vi "Update Status.vi"(7 "Check overlay?":bool, 8 "error in (no error)":errorcluster, 9 "Status":T1=enum."Passed", 10 "Case":string, 11 "Icon Decorator In":refnum<class "Icon Decorator.lvclass">) -> (0 "error out":errorcluster)   [LabVIEW 2020, in "Icon Decorator.lvclass"]
uses:
  Icon Decorator.lvclass
  Core/Result/Status.ctl
  Icon Decorator.lvclass/Icon Decorator.ctl
  <resource>/Framework/Providers/API/mxLvUpdateUI.ctl
  <resource>/Framework/Providers/API/mxLvOverlayState.ctl
  Core/Result/Result.lvlib
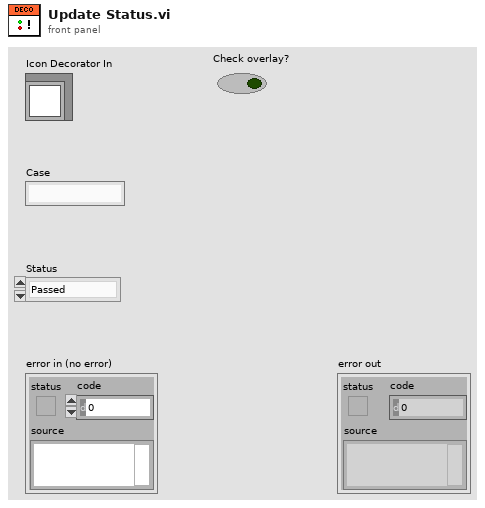
[diagram p1: front panel]
types:
  T1 = typedef "Result.lvlib/Status.ctl" = enum16{"", "Passed", "Failed", "Error", "Skipped", "Setup Error", "Broken", "Teardown Error"}
  T2 = typedef "ItemRef.ctl" = u64
  T3 = typedef "mxLvUpdateUI.ctl" = cluster{"Action":u32, "Optional param 1":string, "Optional param 2":i32, "Optional param 3":string}
  T4 = typedef "mxLvOverlayState.ctl" = cluster{"Overlay Alias":string, "Active":bool}
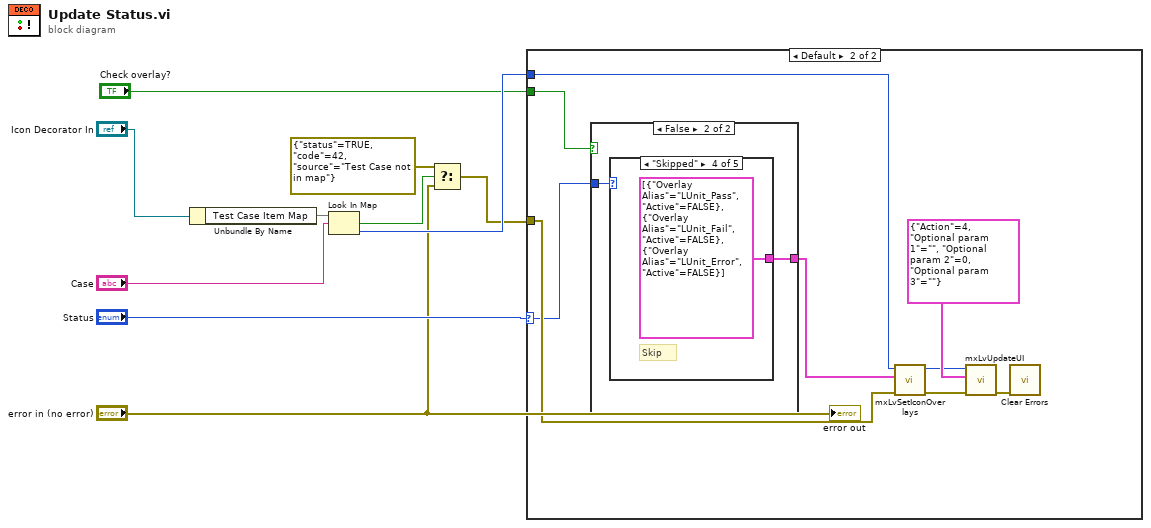
[diagram p0: block diagram]
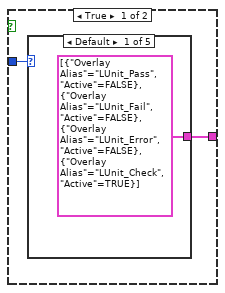
[diagram p3: hidden frame]
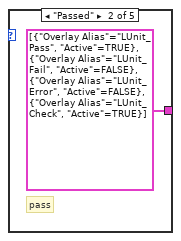
[diagram p4: hidden frame]
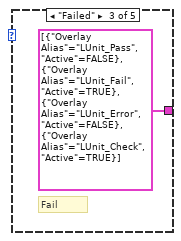
[diagram p5: hidden frame]
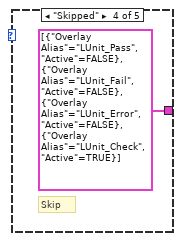
[diagram p6: hidden frame]
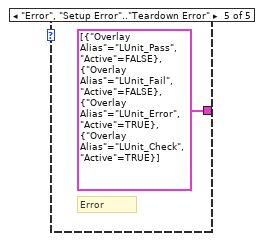
[diagram p7: hidden frame]
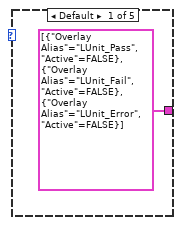
[diagram p8: hidden frame]
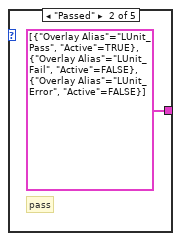
[diagram p9: hidden frame]
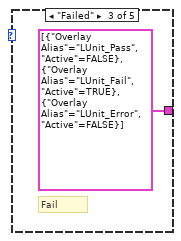
[diagram p10: hidden frame]
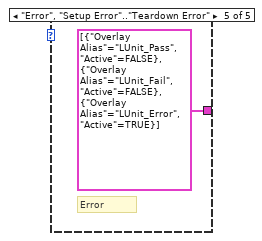
[diagram p11: hidden frame]
diagram:
  n1 = Unbundle By Name("Icon Decorator In") -> ("Test Case Item Map"=w1:map{string, T2})
  n2 = Look In Map(map=w1, key="Case") -> (key not found?=w2:bool, value=w7:T2)  [unwired: 1 in]
  n3 = Select(t=errorcluster {"status"=TRUE, "code"=42, "source"="Test Case not in map"}, s=w2, f="error in (no error)") -> (s? t:f=w6:errorcluster)
  n4 = case shown="Default" "Status" {
    selector: "Status" -> [_ w16]
    tunnel: w7 -> [_ w19]
    tunnel: w6 -> [_ w18]
    tunnel: "Check overlay?" -> [_ w15]
    frame "" {
    }
    frame Default {
      n5 = case shown="False" w15 {
        tunnel: w16 -> [w21 w28]
        tunnel: [w20 w27] -> w14
        frame True {
          n6 = case shown="Default" w21 {
            tunnel: [T4[] [{"Overlay Alias"="LUnit_Pass", "Active"=FALSE}, {"Overlay Alias"="LUnit_Fail", "Active"=FALSE}, {"Overlay Alias"="LUnit_Error", "Active"=FALSE}, {"Overlay Alias"="LUnit_Check", "Active"=TRUE}] ("Array") T4[] [{"Overlay Alias"="LUnit_Pass", "Active"=TRUE}, {"Overlay Alias"="LUnit_Fail", "Active"=FALSE}, {"Overlay Alias"="LUnit_Error", "Active"=FALSE}, {"Overlay Alias"="LUnit_Check", "Active"=TRUE}] ("Array") T4[] [{"Overlay Alias"="LUnit_Pass", "Active"=FALSE}, {"Overlay Alias"="LUnit_Fail", "Active"=TRUE}, {"Overlay Alias"="LUnit_Error", "Active"=FALSE}, {"Overlay Alias"="LUnit_Check", "Active"=TRUE}] ("Array") T4[] [{"Overlay Alias"="LUnit_Pass", "Active"=FALSE}, {"Overlay Alias"="LUnit_Fail", "Active"=FALSE}, {"Overlay Alias"="LUnit_Error", "Active"=FALSE}, {"Overlay Alias"="LUnit_Check", "Active"=TRUE}] ("Array") T4[] [{"Overlay Alias"="LUnit_Pass", "Active"=FALSE}, {"Overlay Alias"="LUnit_Fail", "Active"=FALSE}, {"Overlay Alias"="LUnit_Error", "Active"=TRUE}, {"Overlay Alias"="LUnit_Check", "Active"=TRUE}] ("Array")] -> w20
            frame Default {
            }
            frame "Passed" {
              # "pass"
            }
            frame "Failed" {
              # "Fail"
            }
            frame "Skipped" {
              # "Skip"
            }
            frame "Error", "Setup Error".."Teardown Error" {
              # "Error"
            }
          }
        }
        frame False {
          n7 = case shown="\"Skipped\"" w28 {
            tunnel: [T4[] [{"Overlay Alias"="LUnit_Pass", "Active"=FALSE}, {"Overlay Alias"="LUnit_Fail", "Active"=FALSE}, {"Overlay Alias"="LUnit_Error", "Active"=FALSE}] ("Array") T4[] [{"Overlay Alias"="LUnit_Pass", "Active"=TRUE}, {"Overlay Alias"="LUnit_Fail", "Active"=FALSE}, {"Overlay Alias"="LUnit_Error", "Active"=FALSE}] ("Array") T4[] [{"Overlay Alias"="LUnit_Pass", "Active"=FALSE}, {"Overlay Alias"="LUnit_Fail", "Active"=TRUE}, {"Overlay Alias"="LUnit_Error", "Active"=FALSE}] ("Array") T4[] [{"Overlay Alias"="LUnit_Pass", "Active"=FALSE}, {"Overlay Alias"="LUnit_Fail", "Active"=FALSE}, {"Overlay Alias"="LUnit_Error", "Active"=FALSE}] ("Array") T4[] [{"Overlay Alias"="LUnit_Pass", "Active"=FALSE}, {"Overlay Alias"="LUnit_Fail", "Active"=FALSE}, {"Overlay Alias"="LUnit_Error", "Active"=TRUE}] ("Array")] -> w27
            frame Default {
            }
            frame "Passed" {
              # "pass"
            }
            frame "Failed" {
              # "Fail"
            }
            frame "Skipped" {
              # "Skip"
            }
            frame "Error", "Setup Error".."Teardown Error" {
              # "Error"
            }
          }
        }
      }
      n8 = call <resource>:"mxLvSetIconOverlays.vi"("error in"=w18, "Overlay States"=w14, "Item"=w19) -> ("error out"=w11:errorcluster, "Item"=w12:T2)  [unwired: 7 in]
      n9 = call <resource>:"mxLvUpdateUI.vi"("error in"=w11, "Update UI Settings"=T3 {"Action"=4, "Optional param 1"="", "Optional param 2"=0, "Optional param 3"=""}, "Item"=w12) -> ("error out"=w17:errorcluster)  [unwired: 7 in, 1 out]
      n10 = call <vilib>:"Clear Errors.vi"("error in (no error)"=w17) -> ()  [unwired: 5 in, 2 out]
    }
  }
  "error out" <- "error in (no error)"
